vi "test_VISAInstrument_InitializeSessionsWithUnregisteredSessionsReserved_RemoteSessionsInitialized.vi"(8 "error in":errorcluster) -> (0 "error out":errorcluster, 2 "result":string, 3 "pass":bool)   [LabVIEW 2020, in "MeasurementServerTests.lvlib"]
uses:
  78c0f8c1-8fe2-4936-9d85-28ac64cefb56.vi
  MeasurementServerTests.lvlib
  Runtime/MeasurementLink VISA/MeasurementLink VISA.lvlib
  Runtime/MeasurementLink VISA/Initialize Sessions - NSess.vi
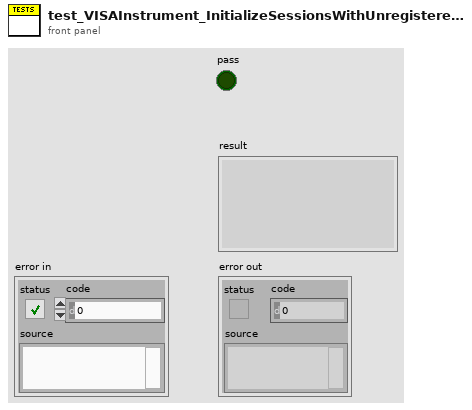
[diagram p1: front panel]
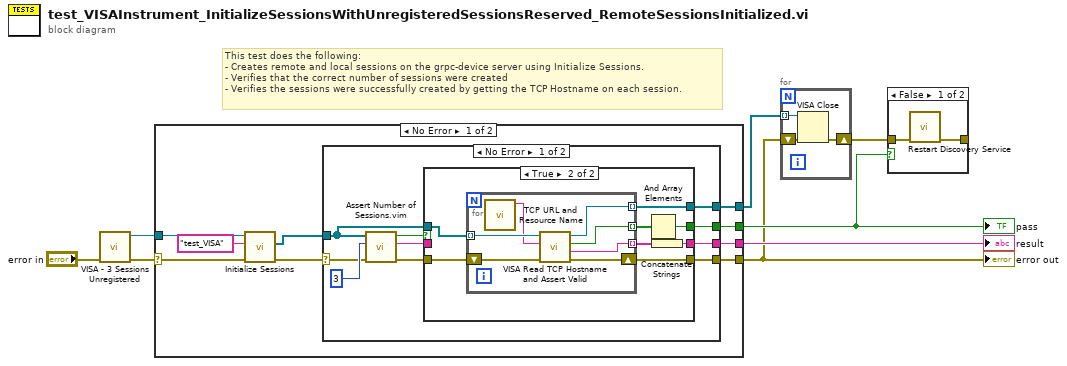
[diagram p0: block diagram]
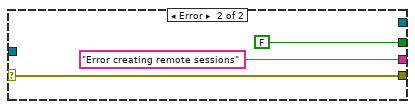
[diagram p3: hidden frame]
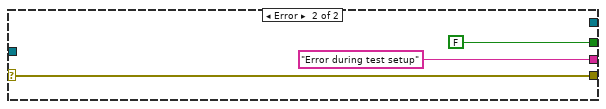
[diagram p4: hidden frame]
diagram:
  # "This test does the following:\n- Creates remote and local sessions on the grpc-device server using Initialize Sessions.\n- Verifies that the correct number of sessions were created\n- Verifies the sessions were successfully created by getting the TCP Hostname on each session."
  n1 = call "VISA - 3 Sessions Unregistered.vi"("error in (no error)"="error in") -> ("error out"=w2:errorcluster, "Session Reservation out"=w1:refnum<class "Session Reservation.lvclass">)  [unwired: 9 in]
  n2 = case shown="No Error" w2 {
    selector: w2 -> [w12 w50]
    tunnel: [w16 w50] -> w4
    tunnel: [w17 FALSE] -> w5
    tunnel: [w15 "Error during test setup" ("f")] -> w8
    tunnel: [w14 _] -> w7
    tunnel: w1 -> [w13 _]
    frame No Error {
      n3 = call-poly "Initialize Sessions.vi"("error in"=w12, "instrument type id"="test_VISA", "session reservation in"=w13) -> ("error out"=w11:errorcluster, "sessions"=w10:refnum<visa-resource-name>[])  [unwired: 5 in, 2 out]
      n4 = case shown="No Error" w11 {
        selector: w11 -> [w21 w48]
        tunnel: [w22 FALSE] -> w17
        tunnel: [w26 w48] -> w16
        tunnel: [w27 "Error creating remote sessions"] -> w15
        tunnel: [w25 _] -> w14
        tunnel: w10 -> [w24 _]
        frame No Error {
          n5 = call "Assert Number of Sessions.vim"("error in"=w21, "expected number of sessions"=3 ("y"), "sessions"=w24) -> ("error out"=w20:errorcluster, "result"=w18:string, "pass"=w19:bool)  [unwired: 6 in]
          n6 = case shown="True" w19 {
            selector: w19 -> [w31 _]
            tunnel: [w30 w33] -> w27
            tunnel: [w29 w37] -> w26
            tunnel: [w28 w36] -> w25
            tunnel: w24 -> [w28 w32]
            tunnel: [w31 w34] -> w22
            tunnel: w20 -> [w29 w35]
            tunnel: w18 -> [w30 _]
            frame False {
            }
            frame True {
              n7 = for {
                tunnel: [w44] -> w39 mode=indexing
                tunnel: [w42] -> w38 mode=indexing
                tunnel: [w43] -> w36 mode=indexing
                tunnel: w32 -> [w45] mode=indexing
                shift-right: [w41] -> w37
                shift-left: w35 -> [w46]
                n8 = call "TCP URL and Resource Name.vi"() -> ("url"=w40:string)  [unwired: 10 in, 1 out]
                n9 = call "VISA Read TCP Hostname and Assert Valid.vi"("error in"=w46, "expected hostname"=w40, "visa refnum in"=w45) -> ("error out"=w41:errorcluster, "result"=w42:string, "pass?"=w44:bool, "visa refnum out"=w43:refnum<visa-resource-name>)  [unwired: 5 in]
              }
              n10 = And Array Elements(Boolean array=w39) -> (logical AND=w34:bool)
              n11 = Concatenate Strings(w38) -> (w33:string)
            }
          }
        }
        frame Error {
        }
      }
    }
    frame Error {
    }
  }
  "error out" <- w4
  "pass" <- w5
  "result" <- w8
  n12 = for {
    tunnel: w7 -> [w55] mode=indexing
    shift-right: [w54] -> w6
    shift-left: w4 -> [w53]
    n13 = VISA Close(VISA resource name=w55, error in (no error)=w53) -> (error out=w54:errorcluster)
  }
  n14 = case shown="False" w5 {
    tunnel: w6 -> [w57 _]
    tunnel: [w56 _] -> _
    frame False {
      n15 = call "Restart Discovery Service.vi"("error in"=w57) -> ("error out"=w56:errorcluster)  [unwired: 10 in]
    }
    frame True {
    }
  }
